vi "Sensor Data Global.vi"(8 "Command":T1, 11 "Transducer Value":u16[](array[numeric])) -> (2 "Sensor Data":T3[](array[typedef]) {"Value" scale=0.0..10.0})   [LabVIEW 2015]
uses:
  Transducer Calibration Display.ctl
  Sensor Enum.ctl
  Thermocouple Data.ctl
  Sensor Data Global Action.ctl
  Sensor Port Mapping Global Action.ctl
  Transducer Calibration Global Action.ctl
panel:
  in  "TC Data":T2[](array[typedef])
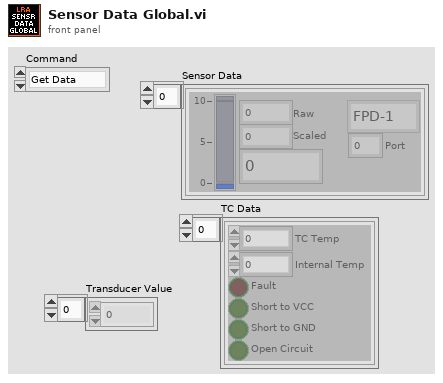
[diagram p1: front panel]
types:
  T1 = typedef "Sensor Data Global Action.ctl" = enum16{"Get Data", "Decode & Store Data"}
  T2 = typedef "Thermocouple Data.ctl" = cluster{"TC Temp":dbl, "Internal Temp":dbl, "Fault":bool, "Short to VCC":bool, "Short to GND":bool, "Open Circuit":bool}
  T3 = typedef "Transducer Calibration Display.ctl" = cluster{"Value":dbl, "Raw":dbl, "Scaled":dbl, "Sensor Name":T4, "Port":u32}
  T4 = typedef "Sensor Enum.ctl" = enum16{"FPD-1", "FPD-2", "FPD-3", "OPD-1", "OPD-2", "OPD-3", "AP-1", "VBAT", "VCOMP", "ICOMP", "TD10"}
  T5 = typedef "Sensor Port Mapping Global Action.ctl" = enum16{"Get", "Set"}
  T6 = typedef "Transducer Calibration Global Action.ctl" = enum16{"Get", "Set"}
  T7 = typedef "Sensor Port Mapping.ctl" = cluster{"Sensor":T4, "Thermocouple?":bool, "Port":u32}
  T8 = typedef "Transducer Calibration Control.ctl" = cluster{"Scale":dbl, "Offset":dbl}
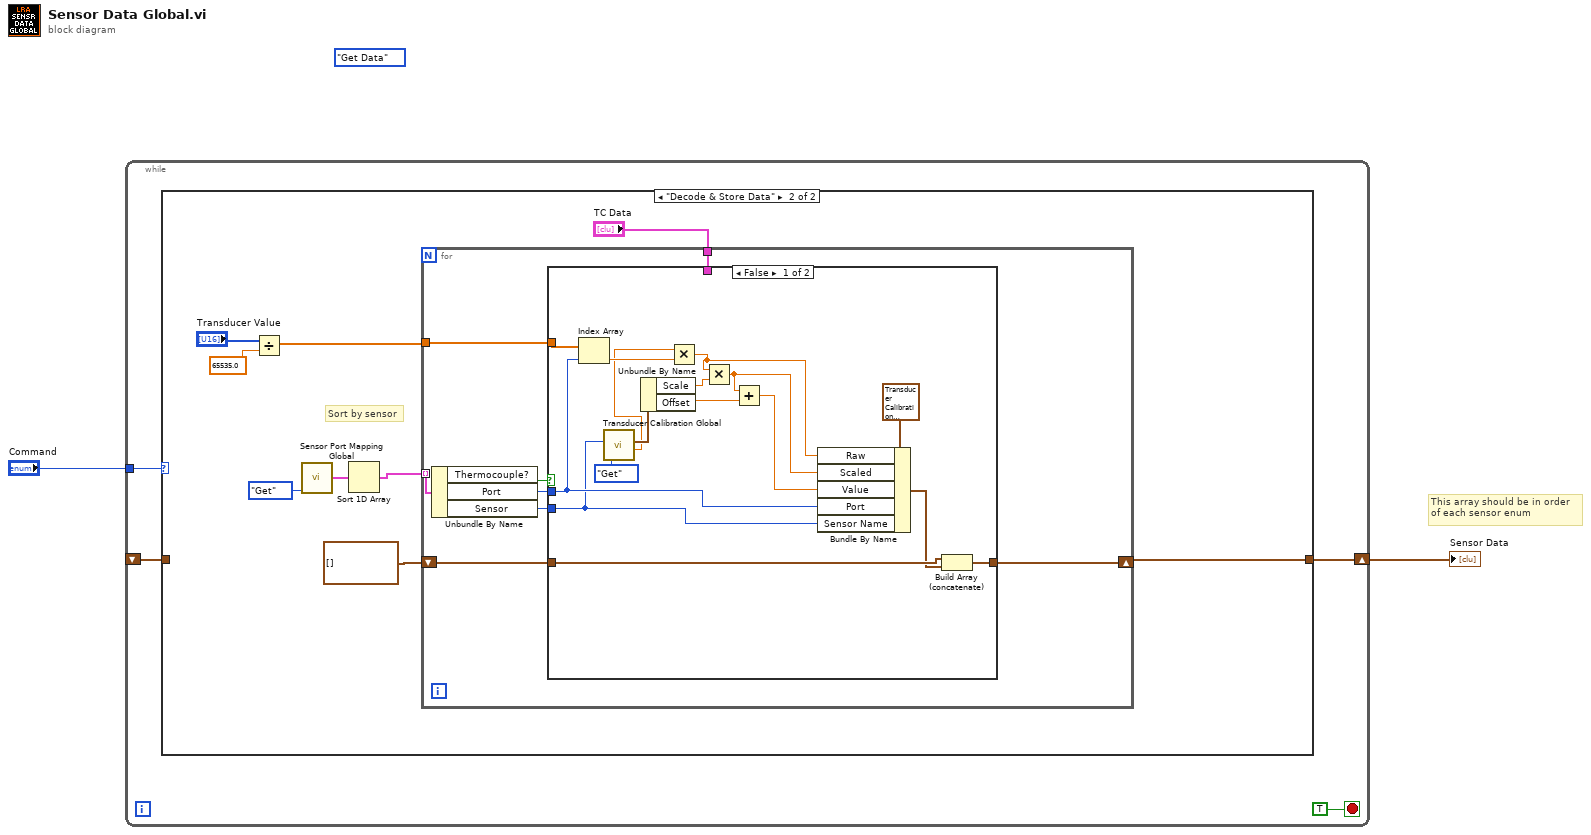
[diagram p0: block diagram]
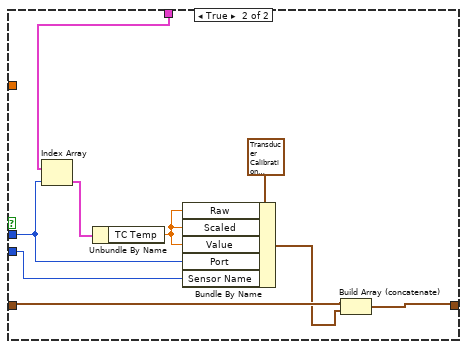
[diagram p3: hidden frame]
diagram:
  (unwired) Sensor_Data_Global_Action."Get Data"
  # "This array should be in order\nof each sensor enum"
  n1 = while {
    shift-right: [w5] -> w2
    shift-left: _ -> [w3]
    tunnel: "Command" -> [w4]
    stop <- TRUE stop-if-true
    n2 = case shown="\"Decode & Store Data\"" w4 {
      tunnel: [w7 w10] -> w5
      tunnel: w3 -> [w7 _]
      frame "Get Data", Default {
      }
      frame "Decode & Store Data" {
        # "Sort by sensor"
        n3 = Divide(x="Transducer Value", y=65535.0) -> (x/y=w13:dbl[])
        n4 = call "Sensor Port Mapping Global.vi"("Action"=Sensor_Port_Mapping_Global_Action."Get") -> ("Mapping List"=w9:T7[])  [unwired: 10 in]
        n5 = Sort 1D Array(array=w9) -> (sorted array=w8:T7[])
        n6 = for {
          tunnel: w8 -> [w24] mode=indexing
          tunnel: w13 -> [w20]
          shift-right: [w18] -> w10
          shift-left: T3[] [] -> [w19]
          tunnel: "TC Data" -> [w17]
          n7 = Unbundle By Name(w24) -> ("Thermocouple?"=w23:bool, "Port"=w22:u32, "Sensor"=w21:T4)
          n8 = case shown="False" w23 {
            tunnel: w22 -> [w36 w45]
            tunnel: w21 -> [w30 w44]
            tunnel: w20 -> [w39 _]
            tunnel: w19 -> [w29 w43]
            tunnel: [w38 w41] -> w18
            tunnel: w17 -> [_ w49]
            frame False {
              n9 = Index Array(array=w39, index=w36) -> (element=w27:dbl)
              n10 = call "Transducer Calibration Global.vi"("Action"=Transducer_Calibration_Global_Action."Get", "Sensor"=w30) -> ("Vref (5V Nominal)"=w25:dbl, "Calibration Data"=w35:T8)  [unwired: 8 in]
              n11 = Unbundle By Name(w35) -> ("Scale"=w34:dbl, "Offset"=w32:dbl)
              n12 = Multiply(x=w25, y=w27) -> (x*y=w26:dbl)
              n13 = Multiply(x=w26, y=w34) -> (x*y=w33:dbl)
              n14 = Add(x=w33, y=w32) -> (x+y=w31:dbl)
              n15 = Bundle By Name(cluster=T3 {"Value"=6.829268292682927, "Raw"=0.0, "Scaled"=0.0, "Sensor Name"=enum."FPD-1", "Port"=0} ("Cluster 3"), "Raw"=w26, "Scaled"=w33, "Value"=w31, "Port"=w36, "Sensor Name"=w30) -> (w28:T3)
              n16 = Build Array (concatenate)(w29, w28) -> (w38:T3[])
            }
            frame True {
              n17 = Index Array(array=w49, index=w45) -> (element=w48:T2)
              n18 = Unbundle By Name(w48) -> ("TC Temp"=w46:dbl)
              n19 = Bundle By Name(cluster=T3 {"Value"=6.829268292682927, "Raw"=0.0, "Scaled"=0.0, "Sensor Name"=enum."FPD-1", "Port"=0} ("Cluster 3"), "Raw"=w46, "Scaled"=w46, "Value"=w46, "Port"=w45, "Sensor Name"=w44) -> (w42:T3)
              n20 = Build Array (concatenate)(w43, w42) -> (w41:T3[])
            }
          }
        }
      }
    }
  }
  "Sensor Data" <- w2
